vi "TwGetSumSpectrumFromH5.vi"(2 "normalize":u8, 3 "spectrum in":dbl[](array[numeric]), 4 "filename":string, 5 "error in (no error)":errorcluster) -> (0 "spectrum out":dbl[](array[numeric]), 1 "error out":errorcluster)   [LabVIEW 2009]
uses:
  TwH5Dll.dll
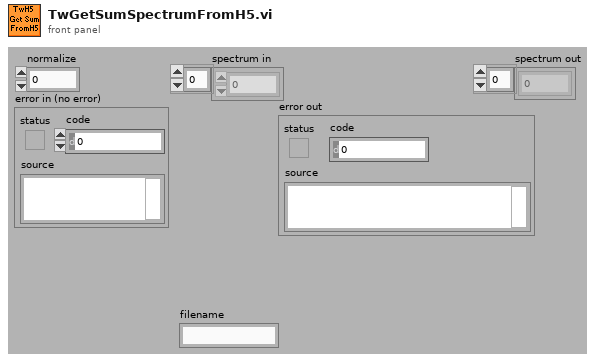
[diagram p1: front panel]
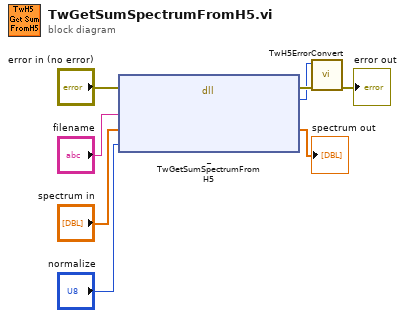
[diagram p0: block diagram]
diagram:
  n1 = dll-call lib="C:/src/85_TofDaq_current/DllWrappers/LabView/TwH5Dll/TwH5Dll.dll" fn="_TwGetSumSpectrumFromH5"(error in="error in (no error)", "filename"="filename", "spectrum"="spectrum in", "normalize"="normalize") -> (error out=w7:errorcluster, "TwRetVal"=w6:i32, "spectrum"=→"spectrum out":dbl[])  [unwired: 4 in, 1 out]
  n2 = call "TwH5ErrorConvert.vi"("error in (no error)"=w7, "error code"=w6) -> ("error out"=→"error out":errorcluster)  [unwired: 9 out]
